vi "UI_Choose String to set Focus.vi"(8 "Error":errorcluster, 9 "Current Index":i32, 10 "Focus Select":T1, 11 "Ref String  Array":refnum<vi>[](array[refnum])) -> (0 "Error Out":errorcluster, 2 "SELECT Out":T1, 3 "String Ref Out":refnum<vi>)   [LabVIEW 2009]
doc: "Chooses the ref and line for focus setting"
uses:
  Controls/Enum/ENUM_Set Focus Select.ctl
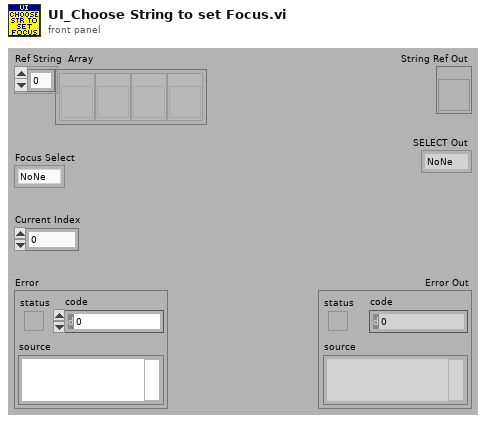
[diagram p1: front panel]
types:
  T1 = typedef "ENUM_Set Focus Select.ctl" = enum16{"NoNe", "Header", "Line 1", "Line 2", "Line 3", "Line 4", "Next", "Back"}
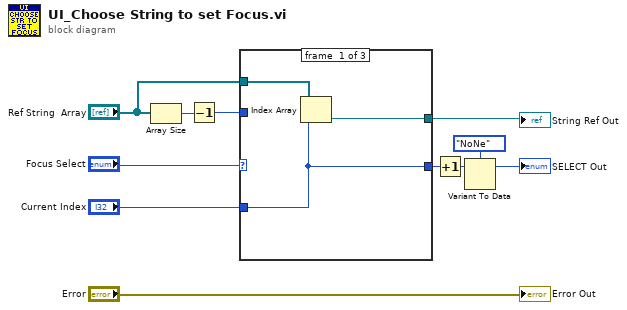
[diagram p0: block diagram]
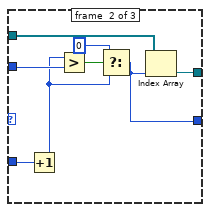
[diagram p2: hidden frame]
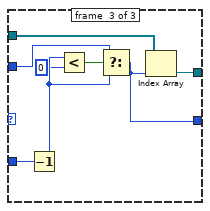
[diagram p3: hidden frame]
diagram:
  n1 = Array Size(array="Ref String  Array") -> (size(s)=w8:i32)
  n2 = Decrement(x=w8) -> (x-1=w9:i32)
  n3 = case shown="\"NoNe\", Default" "Focus Select" {
    tunnel: "Current Index" -> [w12 w20 w28]
    tunnel: w9 -> [_ w19 w25]
    tunnel: "Ref String  Array" -> [w14 w22 w30]
    tunnel: [w13 w21 w29] -> w6
    tunnel: [w12 w15 w23] -> w4
    frame #0 {
      n4 = Index Array(array=w14, index=w12) -> (element=w13:refnum<vi>)
    }
    frame #1 {
      n5 = Increment(x=w20) -> (x+1=w16:i32)
      n6 = Greater?(x=w16, y=w19) -> (0:w18:bool)
      n7 = Select(t=0, s=w18, f=w16) -> (s? t:f=w15:i32)
      n8 = Index Array(array=w22, index=w15) -> (element=w21:refnum<vi>)
    }
    frame #2 {
      n9 = Decrement(x=w28) -> (x-1=w26:i32)
      n10 = Less?(x=w26, y=0) -> (x < y?=w27:bool)
      n11 = Select(t=w25, s=w27, f=w26) -> (s? t:f=w23:i32)
      n12 = Index Array(array=w30, index=w23) -> (element=w29:refnum<vi>)
    }
  }
  "String Ref Out" <- w6
  n13 = Increment(x=w4) -> (x+1=w1:i32)
  n14 = Variant To Data(Variant=w1, type=ENUM_Set_Focus_Select."NoNe" ("Focus Select")) -> (data=→"SELECT Out":T1)  [unwired: 1 in, 1 out]
  "Error Out" <- "Error"
